vi "Curve_Fit_ph.vi"(2 "Bkgnd Value":dbl, 3 "Values In":dbl[](array[numeric]) format="%.4f", 4 "No of points to fit (3)":i32=3, 5 "Positions":dbl[](array[numeric]) format="%.2f") -> (0 "Values Out":dbl[](array[numeric]) format="%.4f", 1 "Polynomial Fit Coefficients":dbl[](array[numeric]) format="%.2f")   [LabVIEW 2010]
uses:
  <vilib>/Analysis/NI_AALPro.lvlib
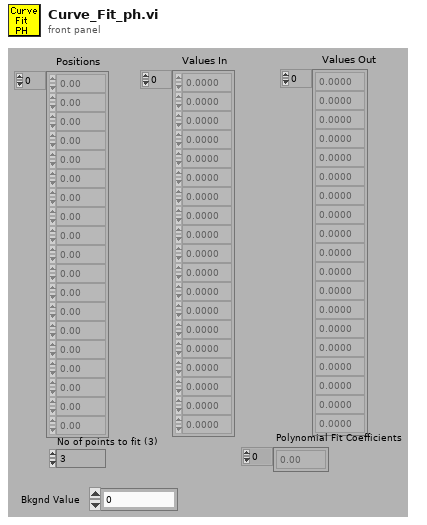
[diagram p1: front panel]
types:
  T1 = enum32{"SVD", "Givens", "Givens2", "Householder", "LU Decomposition", "Cholesky"}
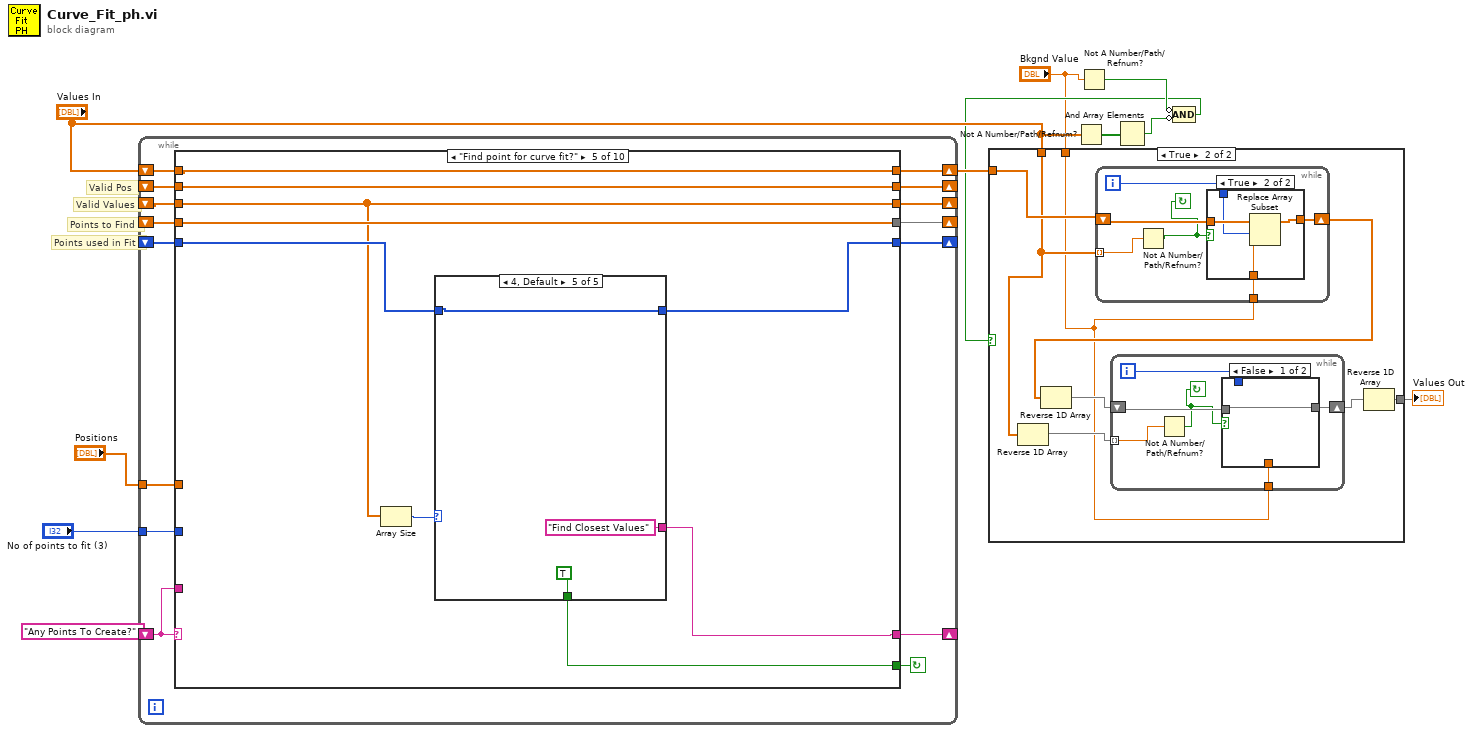
[diagram p0: block diagram]
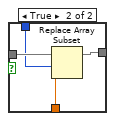
[diagram p3: hidden frame]
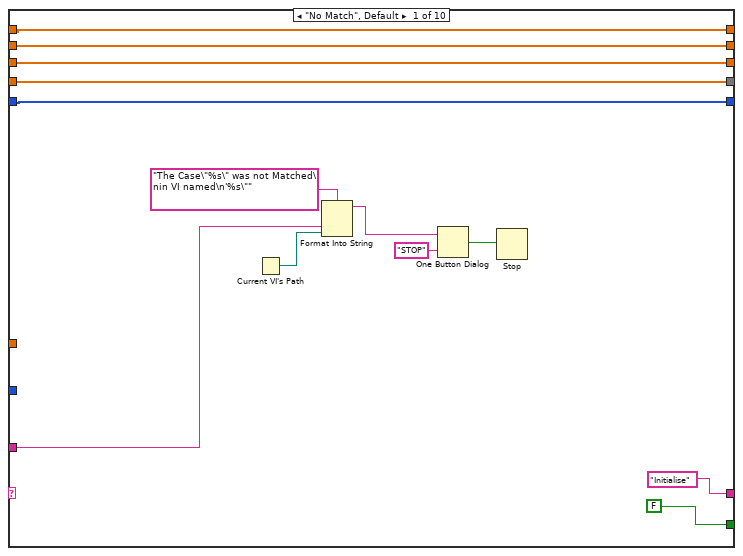
[diagram p5: hidden frame]
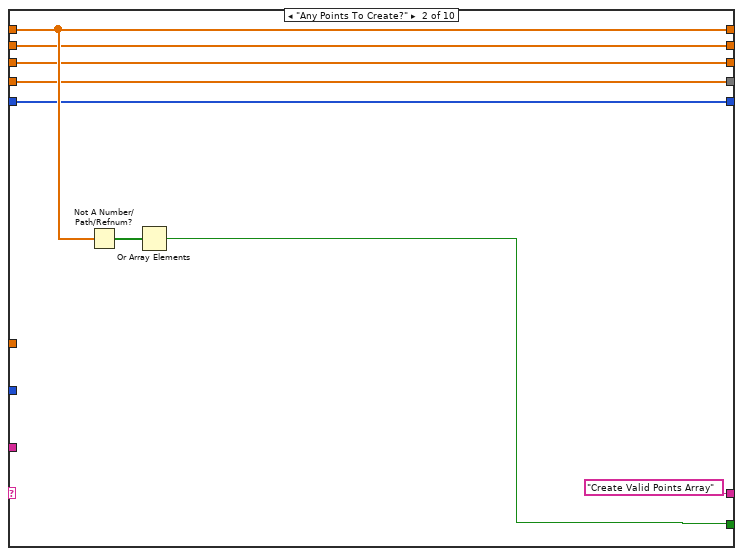
[diagram p6: hidden frame]
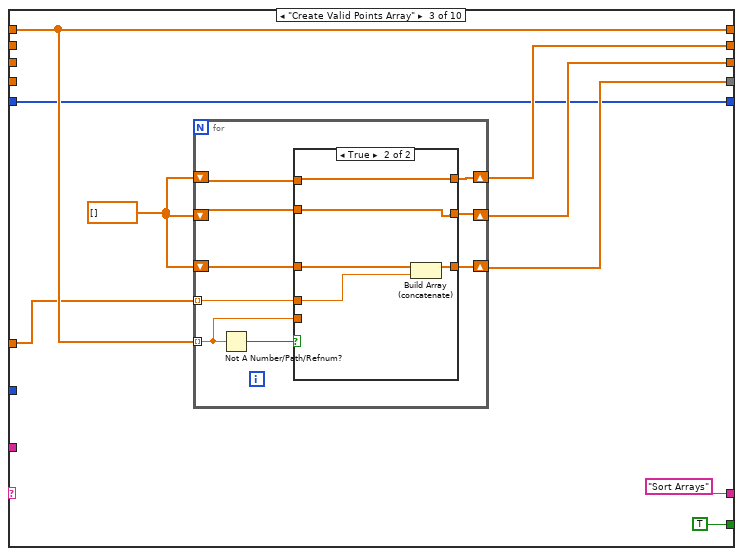
[diagram p7: hidden frame]
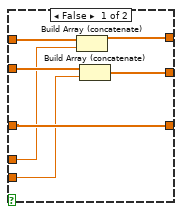
[diagram p8: hidden frame]
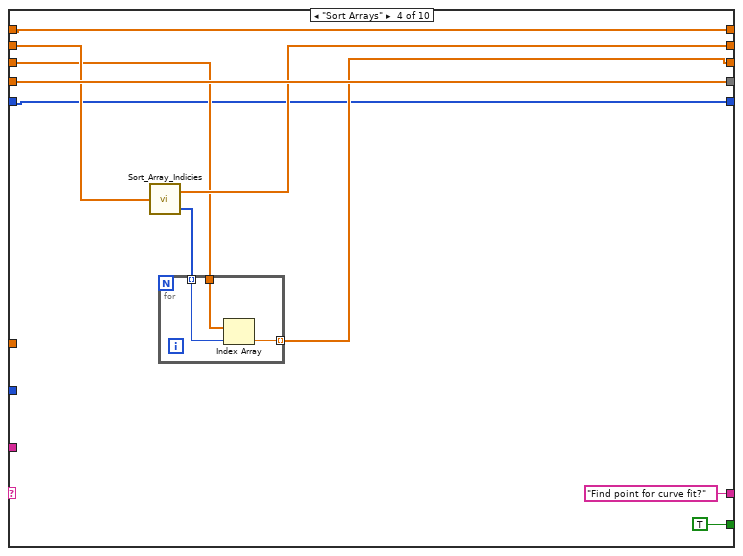
[diagram p9: hidden frame]
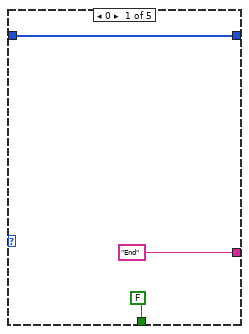
[diagram p10: hidden frame]
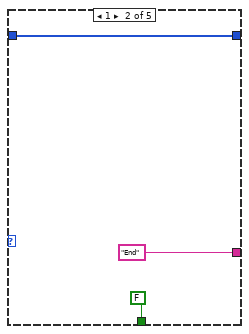
[diagram p11: hidden frame]
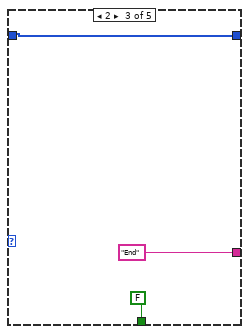
[diagram p12: hidden frame]
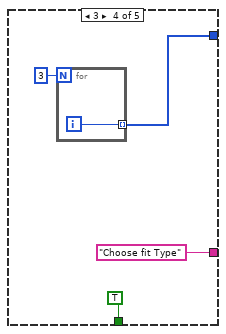
[diagram p13: hidden frame]
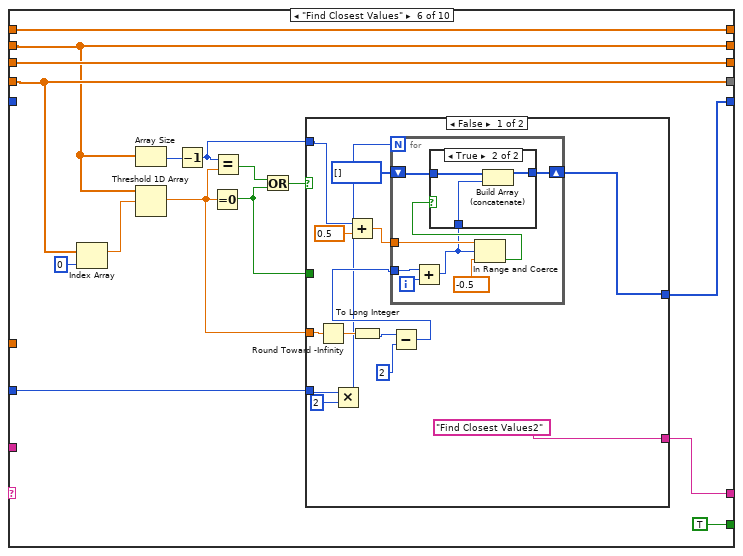
[diagram p14: hidden frame]
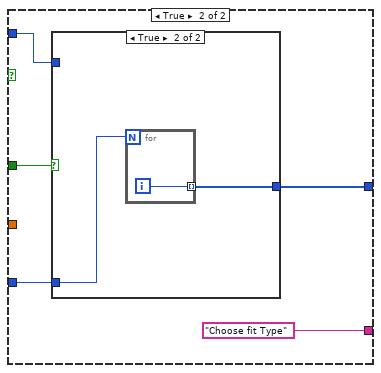
[diagram p16: hidden frame]
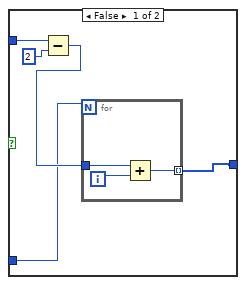
[diagram p17: hidden frame]
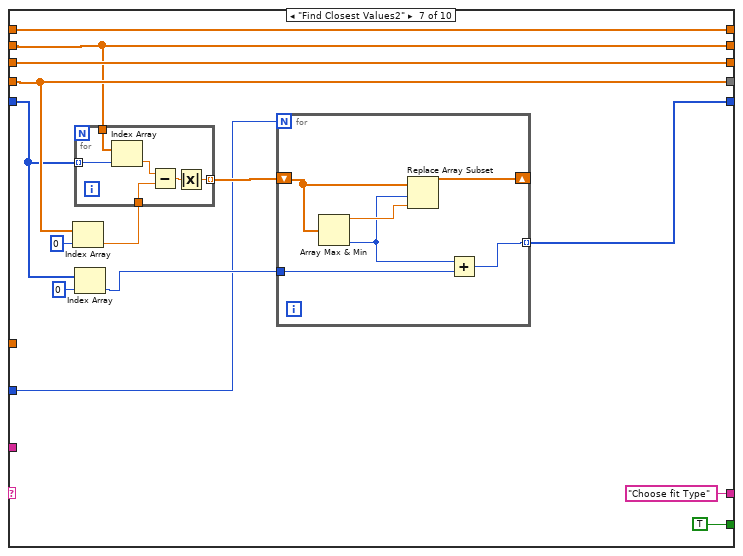
[diagram p18: hidden frame]
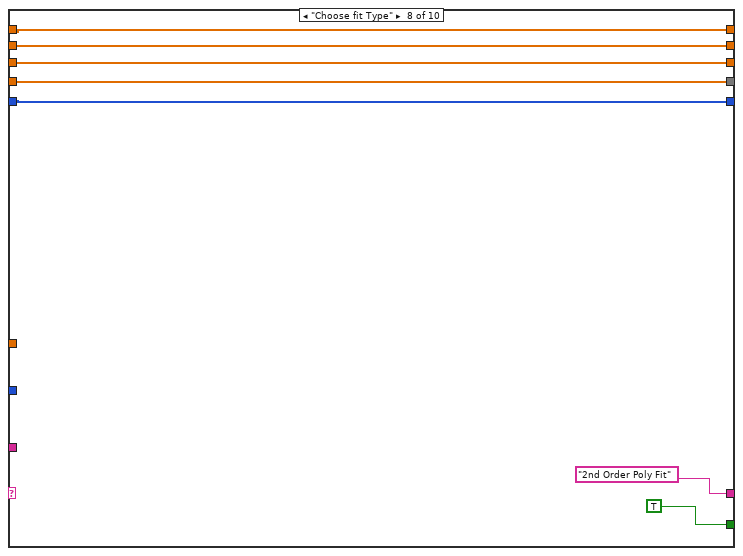
[diagram p19: hidden frame]
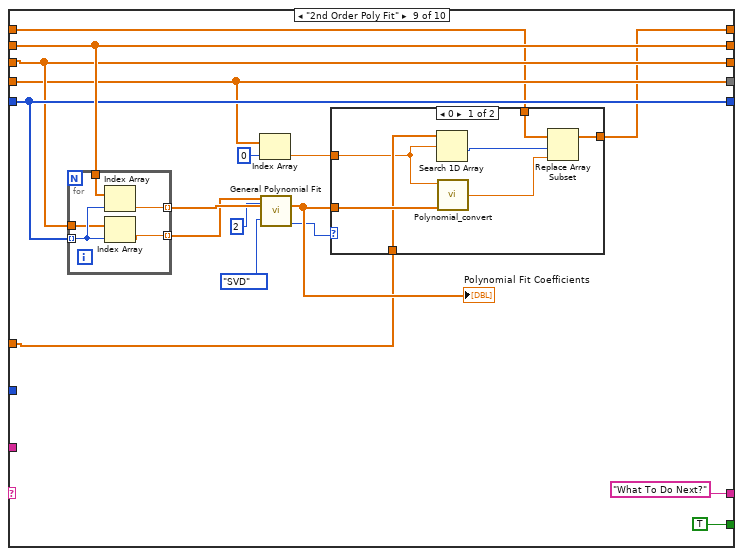
[diagram p20: hidden frame]
diagram:
  # "Points used in Fit"
  # "Valid Values"
  # "Valid Pos"
  # "Points to Find"
  n1 = while {
    shift-left: "Any Points To Create?" -> [w24]
    shift-right: [w25] -> _
    shift-right: [w23] -> w8
    shift-left: "Values In" -> [w22]
    shift-right: [w21] -> _
    shift-left: _ -> [w20]
    tunnel: "Positions" -> [w19]
    shift-right: [w18] -> _
    shift-left: _ -> [w16]
    shift-right: [w17] -> _
    shift-left: _ -> [w15]
    shift-right: [w14] -> _
    shift-left: _ -> [w13]
    tunnel: "No of points to fit (3)" -> [w12]
    stop <- w26 continue-if-true
    n2 = case shown="\"Find point for curve fit?\"" w24 {
      tunnel: [FALSE w44 TRUE TRUE w96 TRUE TRUE TRUE TRUE w239] -> w26
      tunnel: ["Initialise" "Create Valid Points Array" "Sort Arrays" "Find point for curve fit?" w95 w122 "Choose fit Type" "2nd Order Poly Fit" "What To Do Next?" "Find point for curve fit?"] -> w25
      tunnel: w24 -> [w34 _ _ _ _ _ _ _ _ _]
      tunnel: [w31 w46 w55 w87 w99 w132 w188 w205 w210 w243] -> w23
      tunnel: w22 -> [w31 w46 w55 w87 w99 w132 w188 w205 w211 w243]
      tunnel: [w28 w41 w54 w86 w98 w128 w185 w202 w214 w238] -> w21
      tunnel: w20 -> [w28 w41 _ w86 w98 w128 w185 w202 w214 w241]
      tunnel: w19 -> [_ _ w53 _ _ _ _ _ w213 _]
      tunnel: [w30 w43 w50 w84 w92 w127 w183 w204 w223 w244] -> w18
      tunnel: [w29 w42 w49 w82 w91 w130 w186 w203 w221 w245] -> w17
      tunnel: w16 -> [w30 w43 _ w85 w92 w127 w183 w204 w223 w244]
      tunnel: w15 -> [w29 w42 _ w83 w91 w130 w186 w203 w221 w245]
      tunnel: [w27 w40 w48 w81 w94 w123 w180 w201 w222 w246] -> w14
      tunnel: w13 -> [w27 w40 w48 w81 w93 _ w178 w201 w222 w246]
      tunnel: w12 -> [_ _ _ _ _ w117 w175 _ _ _]
      frame "No Match", Default {
        n3 = Current VI's Path() -> (path=w33:path)
        n4 = Format Into String(format string="The Case\"%s\" was not Matched\nin VI named\n'%s\"" ("Format String"), w34, w33) -> (resulting string=w37:string)  [unwired: 2 in, 1 out]
        n5 = One Button Dialog(message=w37, button name ("OK")="STOP") -> (true=w35:bool)
        n6 = Stop(stop? (T)=w35) -> ()
      }
      frame "Any Points To Create?" {
        n7 = Not A Number/Path/Refnum?(number/path/refnum=w46) -> (NaN/Path/Refnum?=w45:bool[])
        n8 = Or Array Elements(Boolean array=w45) -> (logical OR=w44:bool)
      }
      frame "Create Valid Points Array" {
        w51 = dbl[] []
        n9 = for {
          tunnel: w55 -> [w57] mode=indexing
          shift-right: [w63] -> w54
          shift-left: w51 -> [w64]
          tunnel: w53 -> [w62] mode=indexing
          shift-right: [w58] -> w49
          shift-left: w51 -> [w59]
          shift-right: [w60] -> w50
          shift-left: w51 -> [w61]
          n10 = Not A Number/Path/Refnum?(number/path/refnum=w57) -> (NaN/Path/Refnum?=w65:bool)
          n11 = case shown="True" w65 {
            tunnel: w62 -> [w67 w77]
            tunnel: w64 -> [w72 w76]
            tunnel: [w72 w75] -> w63
            tunnel: w61 -> [w71 w74]
            tunnel: [w70 w74] -> w60
            tunnel: w59 -> [w69 w73]
            tunnel: [w68 w73] -> w58
            tunnel: w57 -> [w66 _]
            frame False {
              n12 = Build Array (concatenate)(w71, w67) -> (w70:dbl[])
              n13 = Build Array (concatenate)(w69, w66) -> (w68:dbl[])
            }
            frame True {
              n14 = Build Array (concatenate)(w76, w77) -> (w75:dbl[])
            }
          }
        }
      }
      frame "Sort Arrays" {
        n15 = call "Sort_Array_Indicies.vi"("unsorted array"=w85) -> ("sorted array"=w84:dbl[], "Sort Index"=w78:i32[])
        n16 = for {
          tunnel: w83 -> [w90]
          tunnel: [w89] -> w82 mode=indexing
          tunnel: w78 -> [w88] mode=indexing
          n17 = Index Array(array=w90, index=w88) -> (element=w89:dbl)
        }
      }
      frame "Find point for curve fit?" {
        n18 = Array Size(array=w91) -> (size(s)=w97:i32)
        n19 = case shown="4, Default" w97 {
          tunnel: [FALSE FALSE FALSE TRUE TRUE] -> w96
          tunnel: ["End" "End" "End" "Choose fit Type" "Find Closest Values"] -> w95
          tunnel: [w100 w103 w106 w109 w114] -> w94
          tunnel: w93 -> [w100 w103 w106 _ w114]
          frame 0 {
          }
          frame 1 {
          }
          frame 2 {
          }
          frame 3 {
            n20 = for {
              N: 3 -> [_]
              tunnel: [w113] -> w109 mode=indexing
              i -> [w113]
            }
          }
          frame 4, Default {
          }
        }
      }
      frame "Find Closest Values" {
        n21 = Index Array(array=w128, index=0) -> (element=w129:dbl)
        n22 = Array Size(array=w127) -> (size(s)=w120:i32)
        n23 = Threshold 1D Array(2:w129, 3:w127) -> (0:w121:dbl)  [unwired: 1 out]
        n24 = Decrement(x=w120) -> (x-1=w119:i32)
        n25 = Equal To 0?(x=w121) -> (x = 0?=w124:bool)
        n26 = Equal?(x=w119, y=w121) -> (x = y?=w126:bool)
        n27 = Or(x=w126, y=w124) -> (x .or. y?=w125:bool)
        n28 = case shown="False" w125 {
          tunnel: w124 -> [_ w163]
          tunnel: [w136 w162] -> w123
          tunnel: w119 -> [w140 w161]
          tunnel: ["Find Closest Values2" "Choose fit Type"] -> w122
          tunnel: w121 -> [w145 _]
          tunnel: w117 -> [w135 w159]
          frame False {
            n29 = Round Toward -Infinity(1:w145) -> (0:w144:dbl)
            n30 = Multiply(x=w135, y=2) -> (x*y=w133:i32)
            n31 = Add(x=w140, y=0.5) -> (x+y=w138:dbl)
            n32 = To Long Integer(number=w144) -> (32bit integer=w143:i32)
            n33 = Subtract(x=w143, y=2) -> (x-y=w141:i32)
            n34 = for {
              N: w133 -> [_]
              tunnel: w141 -> [w153]
              shift-right: [w147] -> w136
              shift-left: i32[] [] -> [w149]
              tunnel: w138 -> [w152]
              i -> [w154]
              n35 = Add(x=w153, y=w154) -> (x+y=w148:i32)
              n36 = In Range and Coerce(upper limit=w152, x=w148, lower limit=-0.5) -> (In Range?=w150:bool)  [unwired: 1 out]
              n37 = case shown="True" w150 {
                tunnel: w149 -> [w155 w158]
                tunnel: w148 -> [_ w157]
                tunnel: [w155 w156] -> w147
                frame False {
                }
                frame True {
                  n38 = Build Array (concatenate)(w158, w157) -> (w156:i32[])
                }
              }
            }
          }
          frame True {
            n39 = case shown="True" w163 {
              tunnel: [w168 w173] -> w162
              tunnel: w161 -> [w167 _]
              tunnel: w159 -> [w164 w172]
              frame False {
                n40 = Subtract(x=w167, y=2) -> (x-y=w165:i32)
                n41 = for {
                  N: w164 -> [_]
                  tunnel: [w170] -> w168 mode=indexing
                  tunnel: w165 -> [w169]
                  i -> [w171]
                  n42 = Add(x=w169, y=w171) -> (x+y=w170:i32)
                }
              }
              frame True {
                n43 = for {
                  N: w172 -> [_]
                  tunnel: [w174] -> w173 mode=indexing
                  i -> [w174]
                }
              }
            }
          }
        }
      }
      frame "Find Closest Values2" {
        n44 = Index Array(array=w185, index=0) -> (element=w182:dbl)
        n45 = for {
          tunnel: w178 -> [w194] mode=indexing
          tunnel: w183 -> [w193]
          tunnel: w182 -> [w191]
          tunnel: [w189] -> w181 mode=indexing
          n46 = Index Array(array=w193, index=w194) -> (element=w192:dbl)
          n47 = Subtract(x=w192, y=w191) -> (x-y=w190:dbl)
          n48 = Absolute Value(x=w190) -> (abs(x)=w189:dbl)
        }
        n49 = Index Array(array=w178, index=0) -> (element=w177:i32)
        n50 = for {
          N: w175 -> [_]
          shift-right: [w199] -> _
          shift-left: w181 -> [w200]
          tunnel: [w195] -> w180 mode=indexing
          tunnel: w177 -> [w196]
          n51 = Array Max & Min(array=w200) -> (max value=w198:dbl, min index (indices)=w197:i32)  [unwired: 2 out]
          n52 = Replace Array Subset(array=w200, new element=w198, index=w197) -> (w199:dbl[])
          n53 = Add(x=w197, y=w196) -> (x+y=w195:i32)
        }
      }
      frame "Choose fit Type" {
      }
      frame "2nd Order Poly Fit" {
        n54 = for {
          tunnel: w223 -> [w237]
          tunnel: w222 -> [w236] mode=indexing
          tunnel: w221 -> [w235]
          tunnel: [w234] -> w220 mode=indexing
          tunnel: [w233] -> w219 mode=indexing
          n55 = Index Array(array=w237, index=w236) -> (element=w234:dbl)
          n56 = Index Array(array=w235, index=w236) -> (element=w233:dbl)
        }
        n57 = Index Array(array=w214, index=0) -> (element=w212:dbl)
        n58 = call <vilib>:"General Polynomial Fit.vi"("Y"=w219, "polynomial order"=2, "X"=w220, "algorithm"=T1."SVD") -> ("Polynomial Coefficients"=w216:dbl[], "error"=w209:i32)  [unwired: 8 in, 2 out]
        "Polynomial Fit Coefficients" <- w216
        n59 = case shown="0" w209 {
          tunnel: w216 -> [w231 _]
          tunnel: w213 -> [w230 _]
          tunnel: w212 -> [w229 _]
          tunnel: w211 -> [w228 w232]
          tunnel: [w227 w232] -> w210
          frame 0 {
            n60 = Search 1D Array(1D array=w230, element=w229) -> (index of element=w225:i32)  [unwired: 1 out]
            n61 = call "Polynomial_convert.vi"("Calib constants"=w231, "Voltage"=w229) -> ("Eng Values"=w226:dbl)  [unwired: 4 out]
            n62 = Replace Array Subset(array=w228, new element=w226, index=w225) -> (w227:dbl[])
          }
          frame 1, Default {
          }
        }
      }
      frame "What To Do Next?" {
        n63 = Array Subset(array=w241, index=1) -> (w238:dbl[])  [unwired: 1 in]
        n64 = Array Size(array=w238) -> (size(s)=w240:i32)
        n65 = Greater Than 0?(x=w240) -> (x > 0?=w239:bool)
      }
    }
  }
  n66 = Not A Number/Path/Refnum?(number/path/refnum="Values In") -> (NaN/Path/Refnum?=w6:bool[])
  n67 = Not A Number/Path/Refnum?(number/path/refnum="Bkgnd Value") -> (NaN/Path/Refnum?=w4:bool)
  n68 = And Array Elements(Boolean array=w6) -> (logical AND=w3:bool)
  n69 = Compound Arithmetic op=AND(invert w4, invert w3) -> (w2:bool)
  n70 = case shown="True" w2 {
    tunnel: w8 -> [w248 w256]
    tunnel: "Values In" -> [_ w253]
    tunnel: [w248 w254] -> w5
    tunnel: "Bkgnd Value" -> [_ w249]
    frame False {
    }
    frame True {
      n71 = Reverse 1D Array(array=w253) -> (reversed array=w251:dbl[])
      n72 = while {
        shift-right: [w271] -> w255
        shift-left: w256 -> [w272]
        tunnel: w253 -> [w273] mode=indexing
        tunnel: w249 -> [w270]
        i -> [w269]
        stop <- w268 continue-if-true
        n73 = Not A Number/Path/Refnum?(number/path/refnum=w273) -> (NaN/Path/Refnum?=w268:bool)
        n74 = case shown="True" w268 {
          tunnel: w272 -> [w274 w278]
          tunnel: w269 -> [_ w277]
          tunnel: [w274 w276] -> w271
          tunnel: w270 -> [_ w275]
          frame False {
          }
          frame True {
            n75 = Replace Array Subset(array=w278, new element=w275, index=w277) -> (w276:dbl[])
          }
        }
      }
      n76 = Reverse 1D Array(array=w255) -> (reversed array=w252:dbl[])
      n77 = while {
        shift-right: [w260] -> w250
        shift-left: w252 -> [w261]
        tunnel: w251 -> [w262] mode=indexing
        tunnel: w249 -> [w259]
        i -> [w258]
        stop <- w257 continue-if-true
        n78 = Not A Number/Path/Refnum?(number/path/refnum=w262) -> (NaN/Path/Refnum?=w257:bool)
        n79 = case shown="False" w257 {
          tunnel: w261 -> [w263 w267]
          tunnel: w258 -> [_ w266]
          tunnel: [w263 w265] -> w260
          tunnel: w259 -> [_ w264]
          frame False {
          }
          frame True {
            n80 = Replace Array Subset(array=w267, new element=w264, index=w266) -> (w265:dbl[])
          }
        }
      }
      n81 = Reverse 1D Array(array=w250) -> (reversed array=w254:dbl[])
    }
  }
  "Values Out" <- w5
